vi "saveSetDirectory.vi"() -> (4 "mic":path, 6 "pd":path, 8 "processed":path, 10 "sweeps":path, 15 "crd":path)   [LabVIEW 2011]
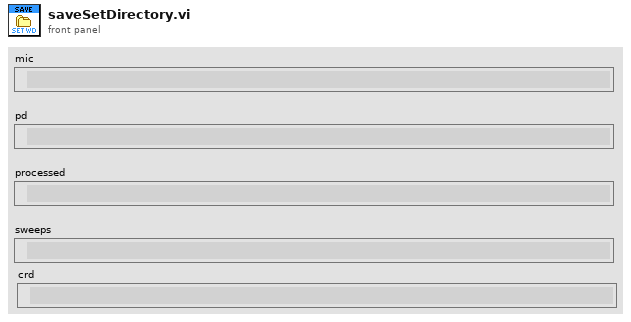
[diagram p1: front panel]
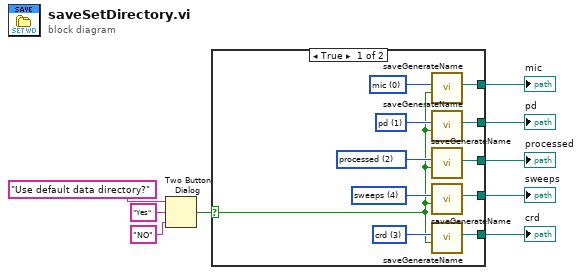
[diagram p0: block diagram]
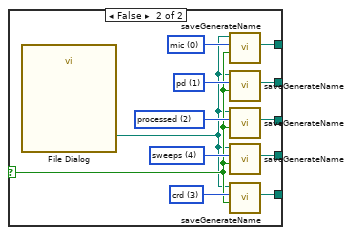
[diagram p2: hidden frame]
diagram:
  n1 = Two Button Dialog(message="Use default data directory?", 1:"NO" ("F button name (\"Cancel\")"), 2:"Yes" ("T button name (\"OK\")")) -> (T button?=w5:bool)
  n2 = case shown="True" w5 {
    selector: w5 -> [w10 w23]
    tunnel: [w16 w25] -> w6
    tunnel: [w15 w26] -> w7
    tunnel: [w14 w27] -> w8
    tunnel: [w13 w28] -> w9
    tunnel: [w11 w21] -> w1
    frame True {
      w12 = u16 3 items=["mic", "pd", "processed", "crd", "sweeps"] ("Type")
      w17 = u16 4 items=["mic", "pd", "processed", "crd", "sweeps"] ("Type")
      w18 = u16 2 items=["mic", "pd", "processed", "crd", "sweeps"] ("Type")
      w19 = u16 1 items=["mic", "pd", "processed", "crd", "sweeps"] ("Type")
      w20 = u16 0 items=["mic", "pd", "processed", "crd", "sweeps"] ("Type")
      n3 = call "saveGenerateName.vi"("use default folder"=w10, "Type"=w20) -> ("file path"=w13:path)  [unwired: 8 in, 1 out]
      n4 = call "saveGenerateName.vi"("use default folder"=w10, "Type"=w19) -> ("file path"=w14:path)  [unwired: 8 in, 1 out]
      n5 = call "saveGenerateName.vi"("use default folder"=w10, "Type"=w18) -> ("file path"=w15:path)  [unwired: 8 in, 1 out]
      n6 = call "saveGenerateName.vi"("use default folder"=w10, "Type"=w17) -> ("file path"=w16:path)  [unwired: 8 in, 1 out]
      n7 = call "saveGenerateName.vi"("use default folder"=w10, "Type"=w12) -> ("file path"=w11:path)  [unwired: 8 in, 1 out]
    }
    frame False {
      w24 = u16 3 items=["mic", "pd", "processed", "crd", "sweeps"] ("Type")
      w29 = u16 4 items=["mic", "pd", "processed", "crd", "sweeps"] ("Type")
      w30 = u16 2 items=["mic", "pd", "processed", "crd", "sweeps"] ("Type")
      w31 = u16 1 items=["mic", "pd", "processed", "crd", "sweeps"] ("Type")
      w32 = u16 0 items=["mic", "pd", "processed", "crd", "sweeps"] ("Type")
      n8 = call "File Dialog"() -> ("selected path"=w22:path)  [unwired: 12 in, 3 out]
      n9 = call "saveGenerateName.vi"("use default folder"=w23, "Type"=w32, "working directory"=w22) -> ("file path"=w28:path)  [unwired: 7 in, 1 out]
      n10 = call "saveGenerateName.vi"("use default folder"=w23, "Type"=w31, "working directory"=w22) -> ("file path"=w27:path)  [unwired: 7 in, 1 out]
      n11 = call "saveGenerateName.vi"("use default folder"=w23, "Type"=w30, "working directory"=w22) -> ("file path"=w26:path)  [unwired: 7 in, 1 out]
      n12 = call "saveGenerateName.vi"("use default folder"=w23, "Type"=w29, "working directory"=w22) -> ("file path"=w25:path)  [unwired: 7 in, 1 out]
      n13 = call "saveGenerateName.vi"("use default folder"=w23, "Type"=w24, "working directory"=w22) -> ("file path"=w21:path)  [unwired: 7 in, 1 out]
    }
  }
  "processed" <- w7
  "pd" <- w8
  "mic" <- w9
  "sweeps" <- w6
  "crd" <- w1
